vi "Get AccessToken.vi"(8 "error in (no error)":errorcluster, 11 "配置":T1={"url"="http://dev.watersystem.com.cn:36091", "loginTokenRequest"={"clientId"="test_client", "clientSecret"="test_secret", "grantType"="password", "password"="59315200", "scope"="read", "userName"="STDTEST001", "userType"="equip"}}) -> (0 "error out":errorcluster, 3 "response":T2)   [LabVIEW 2016, in "opSignIn.lvlib"]
uses:
  <vilib>/httpClient/POSTBuffer.vi
  opSignIn.lvlib
  <vilib>/httpClient/LabVIEWHTTPClient.lvlib
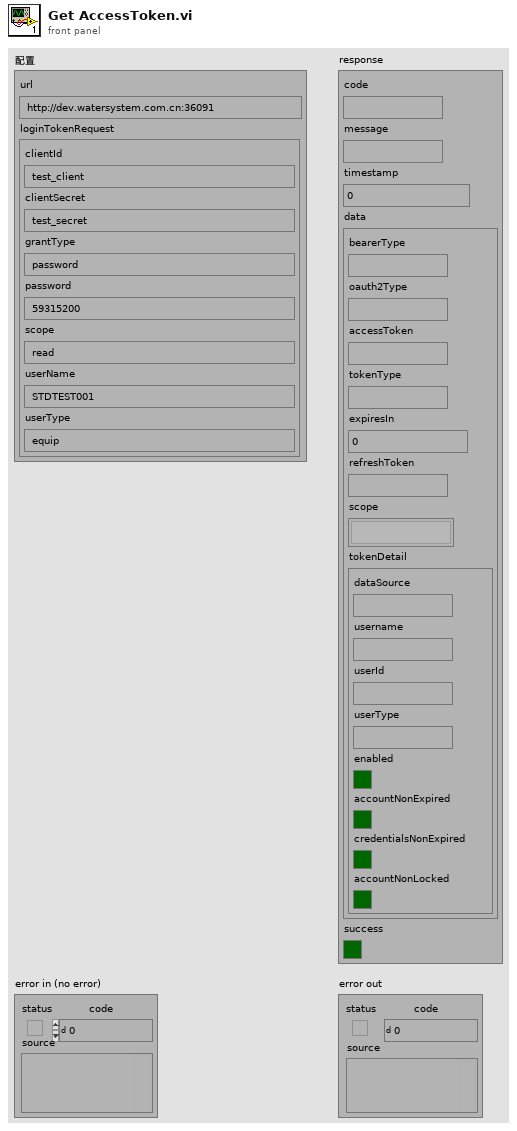
[diagram p1: front panel]
types:
  T1 = cluster{"url":string, "loginTokenRequest":cluster{"clientId":string, "clientSecret":string, "grantType":string, "password":string, "scope":string, "userName":string, "userType":string}}
  T2 = cluster{"code":string, "message":string, "timestamp":u64, "data":cluster{"bearerType":string, "oauth2Type":string, "accessToken":string, "tokenType":string, "expiresIn":u64, "refreshToken":string, "scope":string[], "tokenDetail":cluster{"dataSource":string, "username":string, "userId":string, "userType":string, "enabled":bool, "accountNonExpired":bool, "credentialsNonExpired":bool, "accountNonLocked":bool}}, "success":bool}
  T3 = cluster{"code":string, "message":string, "timestamp":u64, "success":bool}
  T4 = cluster{"clientId":string, "clientSecret":string, "grantType":string, "password":string, "scope":string, "userName":string, "userType":string}
  T5 = typedef "LabVIEWHTTPClient.lvlib/ClientHandle.ctl" = refnum<k1>
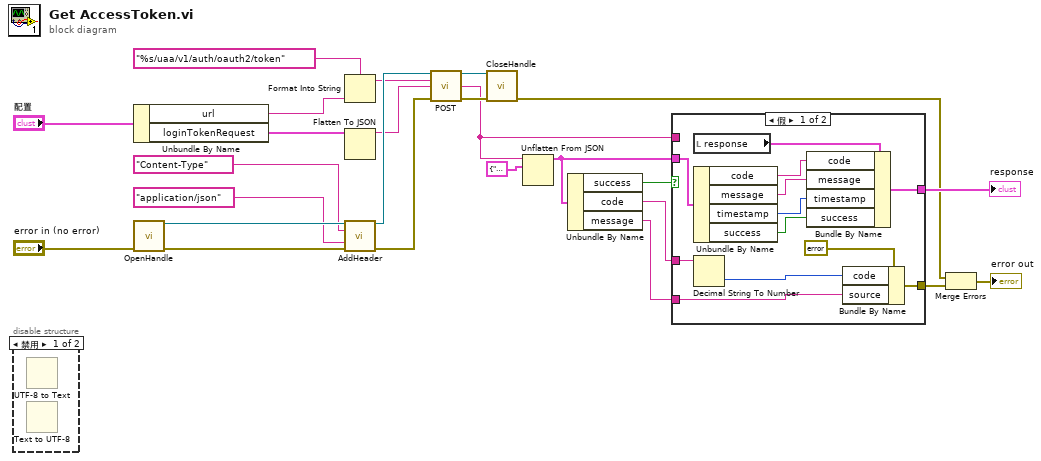
[diagram p0: block diagram]
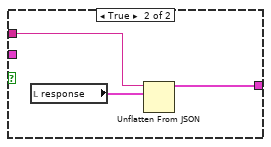
[diagram p2: hidden frame]
diagram:
  n1 = disable-structure shown="禁用" {
    frame Disabled {
      n2 = UTF-8 to Text() -> ()  [unwired: 3 in, 2 out]
      n3 = Text to UTF-8() -> ()  [unwired: 3 in, 2 out]
    }
    frame Enabled {
    }
  }
  n4 = Unbundle By Name("配置") -> ("url"=w11:string, "loginTokenRequest"=w14:T4)
  n5 = call <vilib>:"OpenHandle.vi"("error in (no error)"="error in (no error)") -> ("client handle out"=w25:T5, "error out"=w23:errorcluster)  [unwired: 13 in]
  n6 = Format Into String(format string="%s/uaa/v1/auth/oauth2/token" ("url"), w11) -> (resulting string=w13:string)  [unwired: 2 in, 1 out]
  n7 = Flatten To JSON(anything=w14) -> (JSON string=w17:string)  [unwired: 2 in, 1 out]
  n8 = call <vilib>:"AddHeader.vi"("client handle"=w25, "header"="Content-Type", "value"="application/json", "error in (no error)"=w23) -> ("client handle out"=w21:T5, "error out"=w20:errorcluster)  [unwired: 10 in]
  n9 = call-poly <vilib>:"POST.vi"("client handle"=w21, "url"=w13, "buffer"=w17, "error in (no error)"=w20) -> ("client handle out"=w19:T5, "body"=w7:string, "error out"=w18:errorcluster)  [unwired: 8 in, 1 out]
  n10 = call <vilib>:"CloseHandle.vi"("client handle"=w19, "error in (no error)"=w18) -> ("error out"=w3:errorcluster)  [unwired: 13 in]
  n11 = Unflatten From JSON(JSON string=w7, type and defaults=T3 {"code"="", "message"="", "timestamp"=0, "success"=FALSE} ("response 2")) -> (value=w6:T3)  [unwired: 5 in, 1 out]
  n12 = Unbundle By Name(w6) -> ("success"=w9:bool, "code"=w1:string, "message"=w5:string)
  n13 = case shown="假" w9 {
    tunnel: [w36 w39] -> w8
    tunnel: w7 -> [_ w38]
    tunnel: w6 -> [w35 _]
    tunnel: w5 -> [w29 _]
    tunnel: [w28 _] -> w2
    tunnel: w1 -> [w27 _]
    frame False {
      n14 = local read "response"() -> (w37:T2)
      n15 = Unbundle By Name(w35) -> ("code"=w34:string, "message"=w33:string, "timestamp"=w32:u64, "success"=w31:bool)
      n16 = Decimal String To Number(string=w27) -> (number=w26:i32)  [unwired: 2 in, 1 out]
      n17 = Bundle By Name(cluster=w37, "code"=w34, "message"=w33, "timestamp"=w32, "success"=w31) -> (w36:T2)
      n18 = Bundle By Name(cluster=errorcluster {"status"=TRUE, "code"=0, "source"=""} ("错误常量"), "code"=w26, "source"=w29) -> (w28:errorcluster)
    }
    frame True {
      n19 = local read "response"() -> (w40:T2)
      n20 = Unflatten From JSON(JSON string=w38, type and defaults=w40) -> (value=w39:T2)  [unwired: 5 in, 1 out]
    }
  }
  "response" <- w8
  n21 = Merge Errors(w3, w2) -> (→"error out":errorcluster)
